vi "Select Request.vi"(10 "Output Request":refnum<class "Request.lvclass">, 11 "Input Request":refnum<class "Request.lvclass">) -> (3 "Request":refnum<class "Request.lvclass">)   [LabVIEW 2020, in "HTTP Server.lvlib" / "Server.lvclass"]
uses:
  Server.lvclass
  Server.lvclass/Server.ctl
  <vilib>/IlluminatedG/IG HTTP Utils/HTTP Utils/Request/Request.lvclass
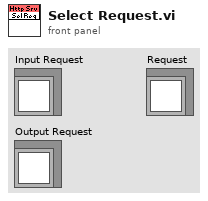
[diagram p1: front panel]
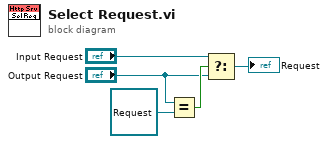
[diagram p0: block diagram]
diagram:
  n1 = Equal?(x="Output Request", y=refnum<class "Request.lvclass"> refnum) -> (x = y?=w5:bool)
  n2 = Select(t="Input Request", s=w5, f="Output Request") -> (s? t:f=→"Request":refnum<class "Request.lvclass">)
